vi "get_stepcount.vi"(8 "error in (no error)":errorcluster, 11 "TCP Network Connection in":refnum<k5>) -> (0 "error out":errorcluster, 2 "Step Count":i32, 3 "TCP Network Connection out":refnum<k5>)   [LabVIEW 2019]
panel:
  out "data out":string
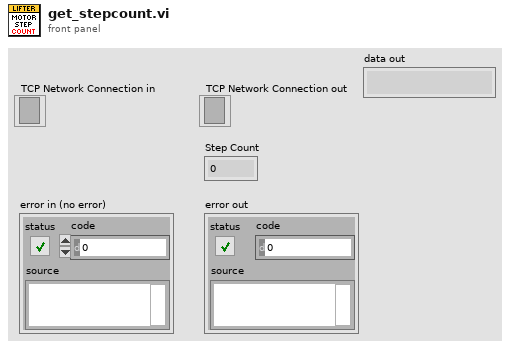
[diagram p1: front panel]
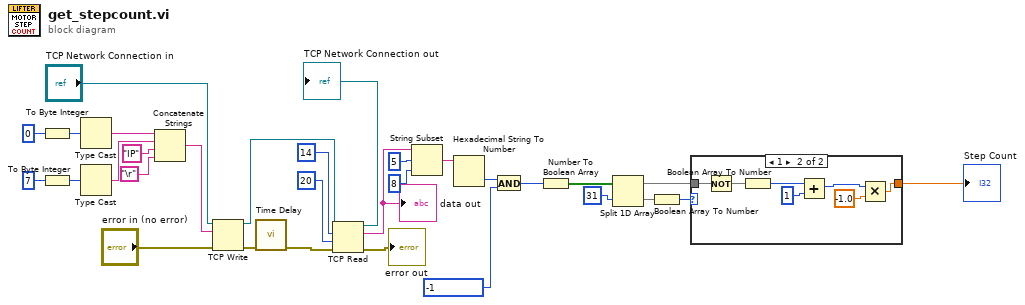
[diagram p0: block diagram]
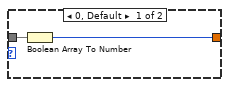
[diagram p2: hidden frame]
diagram:
  n1 = To Byte Integer(number=i8 0) -> (8bit integer=w17:i8)
  n2 = To Byte Integer(number=i8 7) -> (8bit integer=w16:i8)
  n3 = Type Cast(x=w17) -> (*(type *) &x=w23:string)  [unwired: 1 in]
  n4 = Type Cast(x=w16) -> (*(type *) &x=w22:string)  [unwired: 1 in]
  n5 = Concatenate Strings(w23, w22, "IP" ("string"), "\r") -> (w20:string)
  n6 = TCP Write(connection ID="TCP Network Connection in", data in=w20, error in (no error)="error in (no error)") -> (connection ID out=w29:refnum<k5>, error out=w3:errorcluster)  [unwired: 1 in, 1 out]
  n7 = call "Time Delay"("error in (no error)"=w3) -> ("error out"=w2:errorcluster)  [unwired: 10 in]
  n8 = TCP Read(connection ID=w29, bytes to read=14, error in (no error)=w2, 9:20 ("timeout ms (25000)")) -> (connection ID out=→"TCP Network Connection out":refnum<k5>, data out=w30:string, error out=→"error out":errorcluster)  [unwired: 1 in]
  "data out" <- w30
  n9 = String Subset(string=w30, offset (0)=5, length (rest)=8 ("length (rest)")) -> (substring=w31:string)
  n10 = Hexadecimal String To Number(string=w31) -> (number=w15:u32)  [unwired: 2 in, 1 out]
  n11 = And ("Just the \n12 bits")(x=w15, y=-1 ("number")) -> (x .and. y?=w9:u32)
  n12 = Number To Boolean Array(number=w9) -> (Boolean array=w10:bool[])
  n13 = Split 1D Array(array=w10, index=31) -> (first subarray=w13:bool[], second subarray=w11:bool[])
  n14 = Boolean Array To Number(Boolean array=w11) -> (number=w14:u32)
  n15 = case shown="1" w14 {
    tunnel: w13 -> [w33 w40]
    tunnel: [w32 w35] -> w1
    frame 0, Default {
      n16 = Boolean Array To Number(Boolean array=w33) -> (number=w32:u32)
    }
    frame 1 {
      n17 = Not(x=w40) -> (.not. x?=w39:bool[])
      n18 = Boolean Array To Number(Boolean array=w39) -> (number=w37:u32)
      n19 = Add(x=w37, y=u32 1) -> (x+y=w34:u32)
      n20 = Multiply(x=w34, y=-1.0) -> (x*y=w35:dbl)
    }
  }
  "Step Count" <- w1
